vi "Fix Type and Comms to Colour.vi"(9 "Number of sats":u8, 10 "Comms Staus":bool, 11 "Fix Type":u8) -> (2 "3D Fix":bool, 3 "GPS Status":u32)   [LabVIEW 2014]
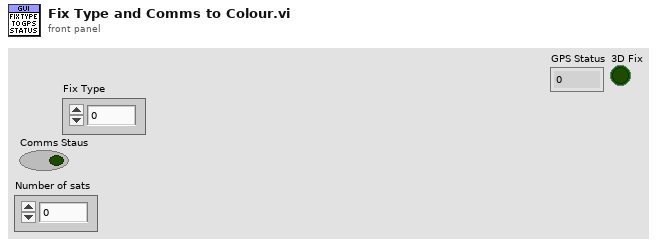
[diagram p1: front panel]
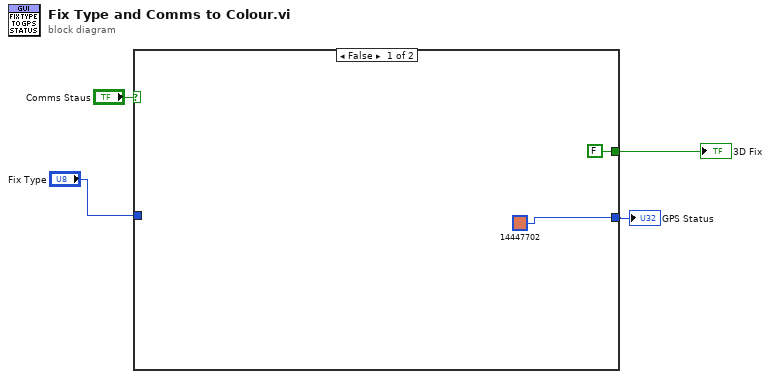
[diagram p0: block diagram]
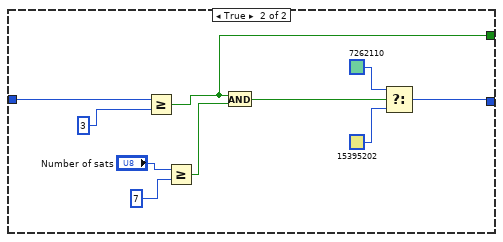
[diagram p2: hidden frame]
diagram:
  n1 = case shown="False" "Comms Staus" {
    tunnel: "Fix Type" -> [_ w14]
    tunnel: [u32 14447702 w15] -> w3
    tunnel: [FALSE w7] -> w1
    frame False {
    }
    frame True {
      n2 = Greater Or Equal?(x=w14, y=u8 3 ("x")) -> (x >= y?=w7:bool)
      n3 = Greater Or Equal?(x="Number of sats", y=u8 7) -> (x >= y?=w9:bool)
      n4 = And(x=w7, y=w9) -> (x .and. y?=w8:bool)
      n5 = Select(t=u32 7262110, s=w8, f=u32 15395202) -> (s? t:f=w15:u32)
    }
  }
  "GPS Status" <- w3
  "3D Fix" <- w1
